vi "Read Voltage.vi"(8 "error in (no error)":errorcluster, 11 "Voltmeter CFG in":refnum<class "Voltmeter CFG.lvclass">) -> (0 "error out":errorcluster, 2 "Voltage":dbl format="%#_g V", 3 "Voltmeter CFG out":refnum<class "Voltmeter CFG.lvclass">)   [LabVIEW 2023, in "PXIe-5172.lvlib" / "Voltmeter CFG.lvclass"]
uses:
  Voltmeter CFG.lvclass
  <vilib>/Analysis/baseanly.llb/Mean (DBL).vi
  <vilib>/Analysis/NI_AALBase.lvlib
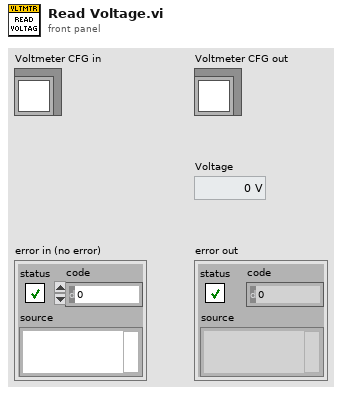
[diagram p1: front panel]
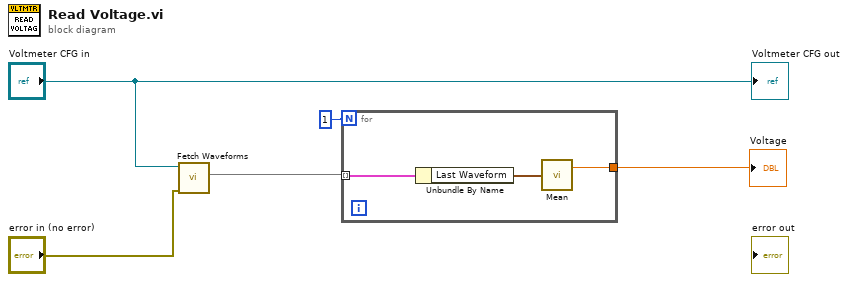
[diagram p0: block diagram]
diagram:
  n1 = call-dynamic "Fetch Waveforms.vi"("error in"="error in (no error)", "object in"="Voltmeter CFG in") -> ("Last Waveforms"=w3:map{u8, waveform(dbl)})  [unwired: 7 in, 2 out]
  n2 = for {
    N: 1 -> [_]
    tunnel: [w8] -> w4
    tunnel: w3 -> [w7] mode=indexing
    n3 = Unbundle By Name(w7) -> ("Last Waveform"=w6:waveform(dbl))
    n4 = call-poly <vilib>:"Mean.vi"("X"=w6) -> ("mean"=w8:dbl)  [unwired: 1 out]
  }
  "Voltage" <- w4
  "Voltmeter CFG out" <- "Voltmeter CFG in"
